vi "Copy.vi"(0 "Conditional in":refnum<class "Conditional.lvclass">, 1 "Linked List Ref":refnum<data-value>, 2 "New Parent ID":string, 5 "Test ID":string, 7 "Insertion Index":i32=-1, 9 "Move?":bool, 11 "error in (no error)":errorcluster, 12 "New ID":string, 13 "Data IDs":variant) -> (3 "Linked List Ref out":refnum<data-value>, 6 "Linked List ID out":string, 14 "Data IDs out":variant, 15 "error out":errorcluster)   [LabVIEW 2017, in "Custom Type Test Executive.lvlib" / "Conditional.lvclass"]
uses:
  <vilib>/gpm_packages/@cs/test-executive/Source/Custom Type Test Executive/Conditional/Conditional.lvclass
  <vilib>/gpm_packages/@cs/linked-list/Source/Linked List/ILinkedList/ILinked List.lvclass
  <vilib>/gpm_packages/@cs/test-executive/Source/Test Executive/Executioner/Executioner.lvclass
  <vilib>/gpm_packages/@cs/data-type-serializer/source/String/String.lvclass/String.ctl
  86d41fb9-efc3-45f2-b7f4-cb2105c1c21b.vi
  607b2b35-f69e-4726-901e-e302bcd403c9.vi
  00ad6bb8-8c6f-43bb-bec9-a9d725405281.vi
  c402d459-f2f3-46d7-992d-5eaaf8c7be91.vi
  <vilib>/gpm_packages/@cs/data-type-serializer/source/String/String.lvclass
  C:/Program Files/National Instruments/LabVIEW 2017/vi.lib/gpm_packages/@cs/data-type-serializer/source/Data Type/Data Type.lvclass
  <vilib>/gpm_packages/@cs/linked-list/Source/Linked List/Linked List Ref/Linked List Ref.lvclass
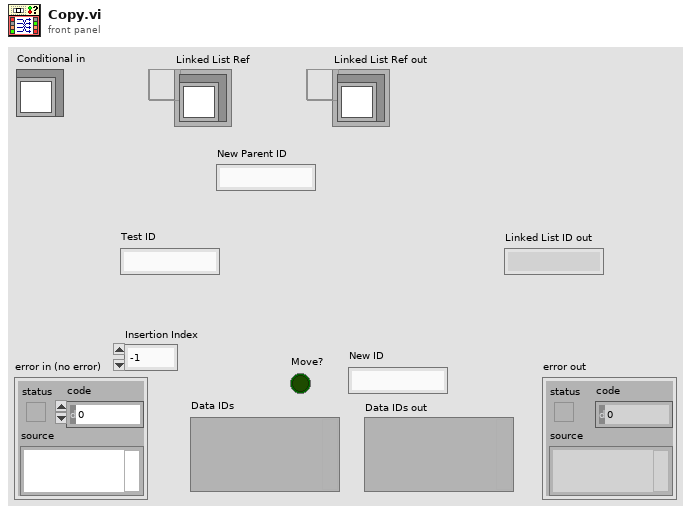
[diagram p1: front panel]
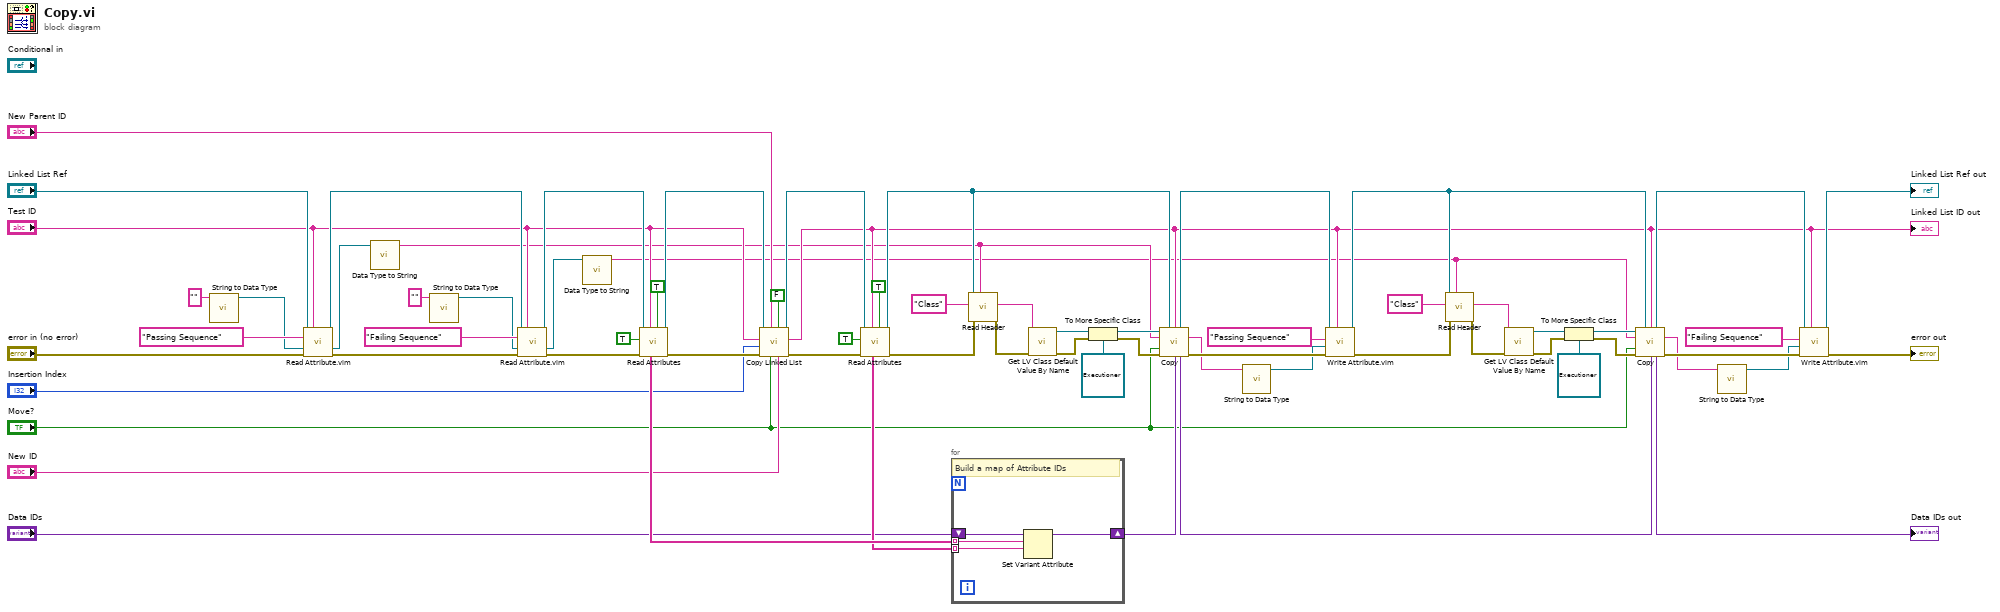
[diagram p0: block diagram]
diagram:
  n1 = call <vilib>:"String to Data Type.vi"("String"="") -> ("Boolean out"=w12:refnum<class "String.lvclass">)  [unwired: 9 in, 1 out]
  n2 = call "Read Attribute.vim"("Linked List Ref"="Linked List Ref", "Linked List ID"="Test ID", "Attribute Name"="Passing Sequence", "Type"=w12, "error in (no error)"="error in (no error)") -> ("Linked List Ref out"=w65:refnum<data-value>, "Attribute"=w10:refnum<class "String.lvclass">, "error out"=w66:errorcluster)  [unwired: 5 in, 3 out]
  n3 = call <vilib>:"Data Type to String.vi"("Data Type"=w10) -> ("String out"=w9:string)  [unwired: 9 in, 1 out]
  n4 = call <vilib>:"String to Data Type.vi"("String"="") -> ("Boolean out"=w7:refnum<class "String.lvclass">)  [unwired: 9 in, 1 out]
  n5 = call "Read Attribute.vim"("Linked List Ref"=w65, "Linked List ID"="Test ID", "Attribute Name"="Failing Sequence", "Type"=w7, "error in (no error)"=w66) -> ("Linked List Ref out"=w29:refnum<data-value>, "Attribute"=w6:refnum<class "String.lvclass">, "error out"=w31:errorcluster)  [unwired: 5 in, 3 out]
  n6 = call <vilib>:"Data Type to String.vi"("Data Type"=w6) -> ("String out"=w5:string)  [unwired: 9 in, 1 out]
  n7 = call <vilib>:"Read Attributes.vi"("Flatten Pointer?"=TRUE, "Linked List ID"="Test ID", "error in (no error)"=w31, "Include Private?"=TRUE, "Linked List Ref"=w29) -> ("error out"=w30:errorcluster, "Linked List Ref out"=w28:refnum<data-value>, "Data IDs"=w26:string[])  [unwired: 1 in, 3 out]
  n8 = call <vilib>:"Copy Linked List.vi"("New Linked List ID"="New ID", "Recursive? (T)"=FALSE, "Move?"="Move?", "New Parent Linked List ID"="New Parent ID", "error in (no error)"=w30, "Insertion Index"="Insertion Index", "Linked List ID"="Test ID", "Linked List Ref"=w28) -> ("error out"=w38:errorcluster, "Linked List ID out"=w13:string, "Linked List Ref out"=w36:refnum<data-value>)  [unwired: 1 out]
  "Linked List ID out" <- w13
  n9 = call <vilib>:"Read Attributes.vi"("Flatten Pointer?"=TRUE, "Linked List ID"=w13, "error in (no error)"=w38, "Include Private?"=TRUE, "Linked List Ref"=w36) -> ("error out"=w37:errorcluster, "Linked List Ref out"=w35:refnum<data-value>, "Data IDs"=w25:string[])  [unwired: 1 in, 3 out]
  n10 = for {
    tunnel: w26 -> [w72] mode=indexing
    tunnel: w25 -> [w71] mode=indexing
    shift-right: [w70] -> w27
    shift-left: "Data IDs" -> [w73]
    # "Build a map of Attribute IDs"
    n11 = Set Variant Attribute(Variant=w73, name=w72, value=w71) -> (Variant out=w70:variant)  [unwired: 1 in, 2 out]
  }
  n12 = call <vilib>:"Read Header.vi"("Linked List ID"=w9, "error in (no error)"=w37, "Header Name"="Class", "Linked List Ref"=w35) -> ("error out"=w61:errorcluster, "Header Value"=w63:string)  [unwired: 4 in, 2 out]
  n13 = call <vilib>:"Get LV Class Default Value By Name.vi"("error in (no error)"=w61, "class name"=w63) -> ("error out"=w60:errorcluster, "object"=w62:refnum<class>)  [unwired: 8 in]
  n14 = To More Specific Class(target class=refnum<class "Executioner.lvclass"> refnum ("Test Executive.lvlib:Executioner.lvclass"), reference=w62, error in=w60) -> (specific class reference=w57:refnum<class "Executioner.lvclass">, error out=w58:errorcluster)
  n15 = call-dynamic "Copy.vi"("Executioner in"=w57, "Linked List Ref"=w35, "New Parent ID"=w13, "Test ID"=w9, "Move?"="Move?", "error in (no error)"=w58, "Data IDs"=w27) -> ("Linked List Ref out"=w54:refnum<data-value>, "Linked List ID out"=w4:string, "Data IDs out"=w34:variant, "error out"=w56:errorcluster)  [unwired: 5 in]
  n16 = call <vilib>:"String to Data Type.vi"("String"=w4) -> ("Boolean out"=w3:refnum<class "String.lvclass">)  [unwired: 9 in, 1 out]
  n17 = call "Write Attribute.vim"("Linked List ID"=w13, "error in (no error)"=w56, "Attribute"=w3, "Attribute Name"="Passing Sequence", "Linked List Ref"=w54) -> ("error out"=w41:errorcluster, "Linked List Ref out"=w42:refnum<data-value>)  [unwired: 3 in, 2 out]
  n18 = call <vilib>:"Read Header.vi"("Linked List ID"=w5, "error in (no error)"=w41, "Header Name"="Class", "Linked List Ref"=w42) -> ("error out"=w46:errorcluster, "Header Value"=w44:string)  [unwired: 4 in, 2 out]
  n19 = call <vilib>:"Get LV Class Default Value By Name.vi"("error in (no error)"=w46, "class name"=w44) -> ("error out"=w47:errorcluster, "object"=w45:refnum<class>)  [unwired: 8 in]
  n20 = To More Specific Class(target class=refnum<class "Executioner.lvclass"> refnum ("Test Executive.lvlib:Executioner.lvclass"), reference=w45, error in=w47) -> (specific class reference=w50:refnum<class "Executioner.lvclass">, error out=w49:errorcluster)
  n21 = call-dynamic "Copy.vi"("Executioner in"=w50, "Linked List Ref"=w42, "New Parent ID"=w13, "Test ID"=w5, "Move?"="Move?", "error in (no error)"=w49, "Data IDs"=w34) -> ("Linked List Ref out"=w53:refnum<data-value>, "Linked List ID out"=w2:string, "Data IDs out"=→"Data IDs out":variant, "error out"=w51:errorcluster)  [unwired: 5 in]
  n22 = call <vilib>:"String to Data Type.vi"("String"=w2) -> ("Boolean out"=w1:refnum<class "String.lvclass">)  [unwired: 9 in, 1 out]
  n23 = call "Write Attribute.vim"("Linked List ID"=w13, "error in (no error)"=w51, "Attribute"=w1, "Attribute Name"="Failing Sequence", "Linked List Ref"=w53) -> ("error out"=→"error out":errorcluster, "Linked List Ref out"=→"Linked List Ref out":refnum<data-value>)  [unwired: 3 in, 2 out]
